vi "Generate Test Data.vi"(11 "Single in":refnum<class "Single.lvclass">) -> (3 "Single out":refnum<class "Single.lvclass">)   [LabVIEW 2014, in "Base Data Class.lvlib" / "Single.lvclass"]
uses:
  Single.lvclass
  Single.lvclass/Single.ctl
  Data.lvclass
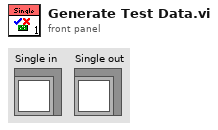
[diagram p1: front panel]
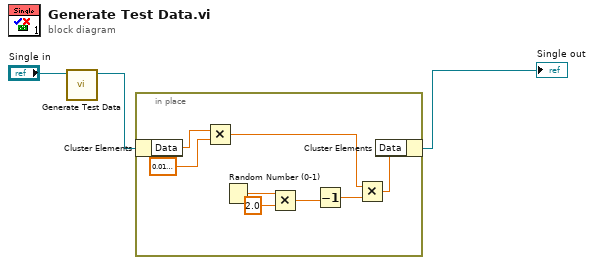
[diagram p0: block diagram]
diagram:
  n1 = call-parent "Generate Test Data.vi"("Data in"="Single in") -> ("Data out"=w2:refnum<class "Single.lvclass">)  [unwired: 10 in]
  n2 = in-place {
    n3 = in-place-cluster #1(w2) -> ("Data"=w5:sgl)
    n4 = Multiply(x=w5, y=sgl 0.02) -> (x*y=w6:sgl)
    n5 = Random Number (0-1)() -> (number: 0 to 1=w10:dbl)
    n6 = Multiply(x=w10, y=2.0) -> (x*y=w8:dbl)
    n7 = Decrement(x=w8) -> (x-1=w7:dbl)
    n8 = Multiply(x=w6, y=w7) -> (x*y=w4:dbl)
    n9 = in-place-cluster #1("Data"=w4) -> (→"Single out":refnum<class "Single.lvclass">)
  }
